vi "Set Timeout.vi"(7 "nats connection in":T1, 11 "timeout ms in":i32) -> (3 "timeout ms out":i32)   [LabVIEW 2013, in "NATS Core.lvlib"]
doc: "If input of timeout is -2 then use the timeout defined in the nats connection input."
uses:
  NATS Core.lvlib
  Controls/nats connection.ctl
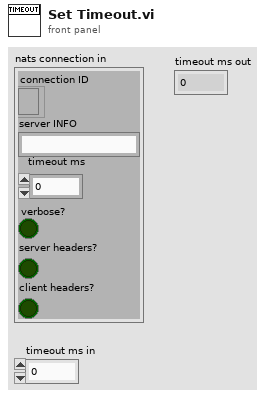
[diagram p1: front panel]
types:
  T1 = typedef "NATS Core.lvlib/nats connection.ctl" = cluster{"connection ID":refnum<k5>, "server INFO":string, "timeout ms":i32, "verbose?":bool, "server headers?":bool, "client headers?":bool}
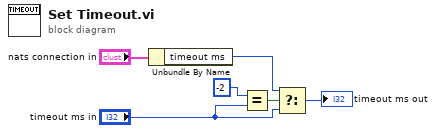
[diagram p0: block diagram]
diagram:
  n1 = Unbundle By Name("nats connection in") -> ("timeout ms"=w5:i32)
  n2 = Equal?(x=-2, y="timeout ms in") -> (x = y?=w2:bool)
  n3 = Select(t=w5, s=w2, f="timeout ms in") -> (s? t:f=→"timeout ms out":i32)
